vi "Create Listener.vi"(8 "error in (no error)":errorcluster, 10 "Timeout ms (25000)":i32, 11 "TCP Server in":refnum<class "TCP Server.lvclass">) -> (0 "error out":errorcluster, 3 "TCP Server out":refnum<class "TCP Server.lvclass">)   [LabVIEW 2017, in "TCP Interface.lvlib" / "TCP Server.lvclass"]
uses:
  <vilib>/gpm_packages/@cs/Network-sink/Source/TCP Interface/TCP Server/TCP Server.lvclass
  <vilib>/gpm_packages/@cs/Network-sink/Source/TCP Interface/TCP Server/TCP Server.lvclass/TCP Server.ctl
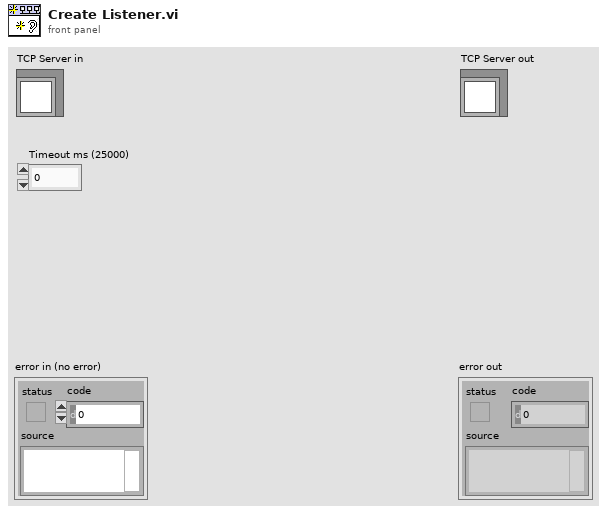
[diagram p1: front panel]
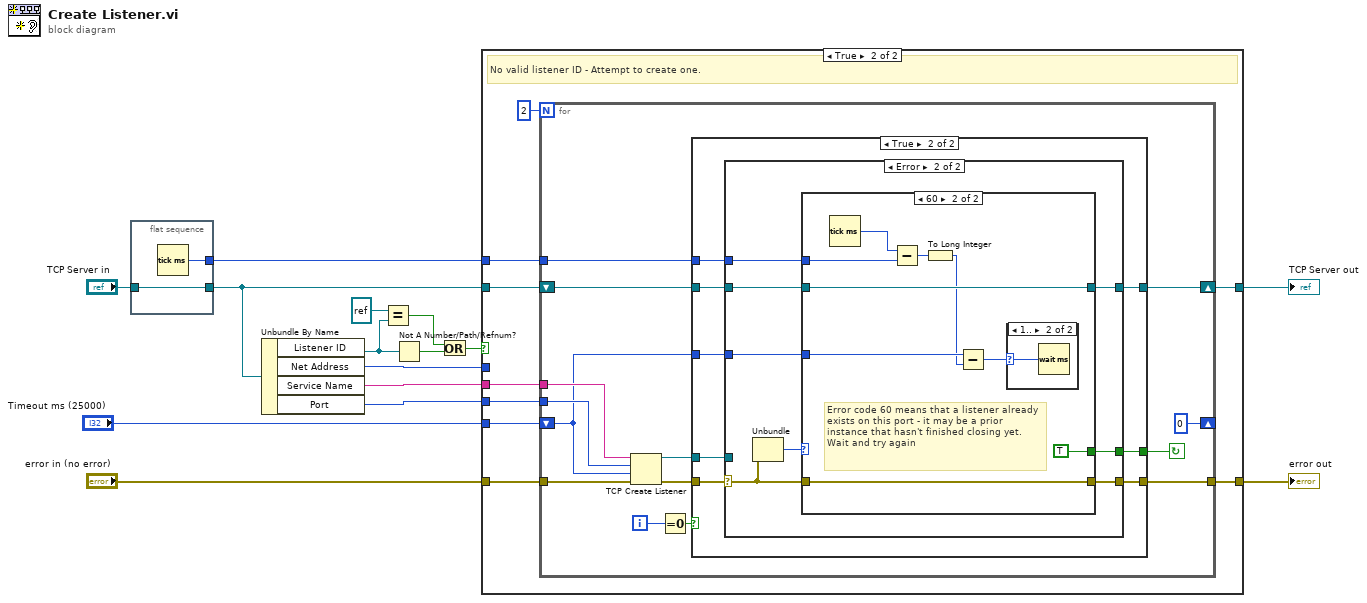
[diagram p0: block diagram]
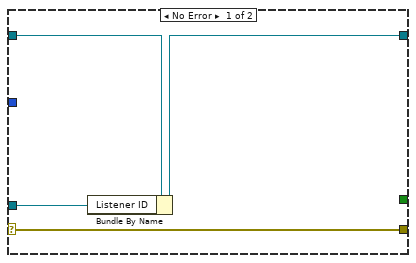
[diagram p4: hidden frame]
diagram:
  n1 = flat-sequence {
    tunnel: [w17] -> w3
    tunnel: "TCP Server in" -> [w17]
    tunnel: [w16] -> w1
    frame #0 {
      n2 = Tick Count (ms)() -> (millisecond timer value=w16:u32)
    }
  }
  n3 = Unbundle By Name(w3) -> ("Listener ID"=w8:refnum<k5>, "Net Address"=w12:u32, "Service Name"=w11:string, "Port"=w10:u16)
  n4 = Equal?(x=refnum<k5> refnum, y=w8) -> (x = y?=w6:bool)
  n5 = Not A Number/Path/Refnum?(number/path/refnum=w8) -> (NaN/Path/Refnum?=w9:bool)
  n6 = Or(x=w6, y=w9) -> (x .or. y?=w5:bool)
  n7 = case shown="True" w5 {
    tunnel: "error in (no error)" -> [w18 w28]
    tunnel: [w18 w23] -> w14
    tunnel: "Timeout ms (25000)" -> [_ w21]
    tunnel: w12 -> [_ _]
    tunnel: w11 -> [_ w27]
    tunnel: w10 -> [_ w26]
    tunnel: w3 -> [w19 w25]
    tunnel: [w19 w24] -> w4
    tunnel: w1 -> [_ w22]
    frame False {
      # "Already have a valid listener ID - don't create another"
    }
    frame True {
      # "No valid listener ID - Attempt to create one."
      n8 = for {
        N: 2 -> [_]
        tunnel: w27 -> [w41]
        tunnel: w26 -> [w40]
        tunnel: w22 -> [w34]
        shift-right: [w38] -> w24
        shift-left: w25 -> [w39]
        shift-right: [0 ("Timeout ms (25000)")] -> _
        shift-left: w21 -> [w33]
        tunnel: w28 -> [w42]
        tunnel: [w35] -> w23
        i -> [w30]
        stop <- w31 continue-if-true
        n9 = TCP Create Listener(8:w42, 9:w33, 10:w40, 11:w41) -> (0:w37:errorcluster, 3:w36:refnum<k5>)  [unwired: 1 in, 1 out]
        n10 = Equal To 0?(x=w30) -> (x = 0?=w29:bool)
        n11 = case shown="True" w29 {
          tunnel: w39 -> [w44 w52]
          tunnel: [w44 w51] -> w38
          tunnel: w37 -> [w43 w50]
          tunnel: w36 -> [_ w49]
          tunnel: [w43 w48] -> w35
          tunnel: w34 -> [_ w47]
          tunnel: w33 -> [_ w46]
          tunnel: [_ w45] -> w31
          frame False {
          }
          frame True {
            n12 = case shown="Error" w50 {
              selector: w50 -> [w55 w64]
              tunnel: w52 -> [w56 w62]
              tunnel: [w54 w61] -> w51
              tunnel: w49 -> [w53 _]
              tunnel: [w55 w59] -> w48
              tunnel: w47 -> [_ w60]
              tunnel: w46 -> [_ w58]
              tunnel: [_ w57] -> w45
              frame No Error {
                n13 = Bundle By Name(cluster=w56, "Listener ID"=w53) -> (w54:refnum<class "TCP Server.lvclass">)
              }
              frame Error {
                n14 = Unbundle(w64) -> ("code"=w63:i32)  [unwired: 2 out]
                n15 = case shown="60" w63 {
                  tunnel: w64 -> [w65 w68]
                  tunnel: w62 -> [w66 w75]
                  tunnel: [w66 w75] -> w61
                  tunnel: w60 -> [_ w73]
                  tunnel: [w65 w68] -> w59
                  tunnel: w58 -> [_ w71]
                  tunnel: [_ TRUE] -> w57
                  frame 0, Default {
                  }
                  frame 60 {
                    # "Error code 60 means that a listener already exists on this port - it may be a prior instance that hasn't finished closing yet. Wait and try again"
                    n16 = Tick Count (ms)() -> (millisecond timer value=w74:u32)
                    n17 = Subtract(x=w74, y=w73) -> (x-y=w72:u32)
                    n18 = To Long Integer(number=w72) -> (32bit integer=w67:i32)
                    n19 = Subtract(x=w71, y=w67) -> (x-y=w70:i32)
                    n20 = case shown="1.." w70 {
                      selector: w70 -> [_ w76]
                      frame 0, Default {
                      }
                      frame 1.. {
                        n21 = Wait (ms)(milliseconds to wait=w76) -> ()  [unwired: 1 out]
                      }
                    }
                  }
                }
              }
            }
          }
        }
      }
    }
  }
  "error out" <- w14
  "TCP Server out" <- w4
